vi "sv_Get Audio Weighting Filter Coefficients.vi"(6 "reset filter (F)":bool, 8 "error in (no error)":errorcluster, 9 "weighting filter":T2 items=["Linear", "A-weighting", "B-weighting", "C-weighting", "ITU-R 468-4", "Dolby", "CCITT", "C-message", "Wb", "Wc", "Wd", "We", "Wf", "Wh", "Wj", "Wk", "Wm", "AES17 20 kHz lowpass", "AES17 40 kHz lowpass", "AES17 20 kHz highpass", "AES17 40 kHz highpass"], 11 "scaled signal":waveform(dbl)={"t0"=timestamp(0 s since 1904-01-01), "dt"=0.0, "Y"=[]}) -> (0 "error out":errorcluster, 2 "filter coefficients":T1 {"Forward Coefficients" format="%.4f"; "Reverse Coefficients" format="%.4f"}, 3 "dup scaled signal":waveform(dbl))   [LabVIEW 2017]
doc: "Designs the A, B, or C weighting filter coefficients. The design is based on the ANSI S1.42-1986 standard. This VI also returns the maximum frequency, expressed in hertz, within the tolerance limits based on the selected type (Type 1 or Type 0), according to the ANSI S1.4-1986 standard."
uses:
  <vilib>/addons/_NISVFA/_Shared subVIs/Controls/svc_Weighting Filter Text Ring.ctl
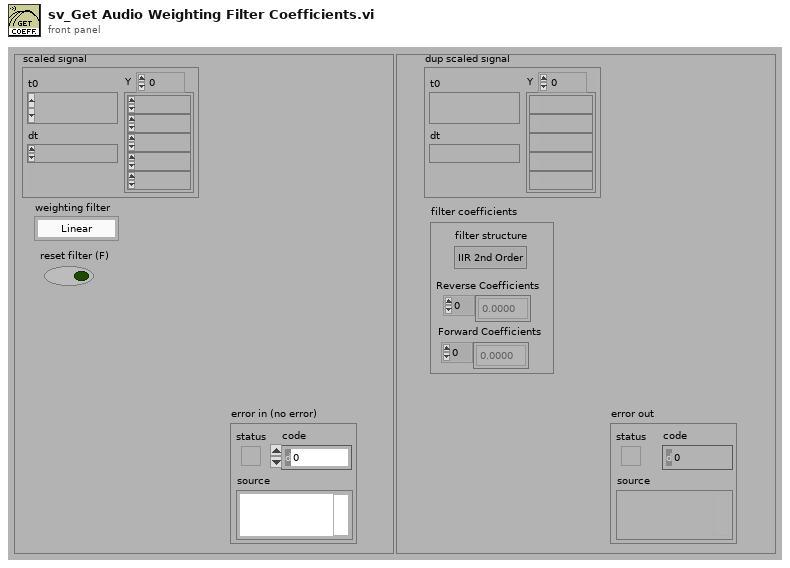
[diagram p1: front panel]
types:
  T1 = cluster{"filter structure":enum32{"IIR 2nd Order", "IIR 4th Order"}, "Reverse Coefficients":dbl[], "Forward Coefficients":dbl[]}
  T2 = typedef "svc_Weighting Filter Text Ring.ctl" = u16
  T3 = cluster{"filter structure":enum32{"IIR 2nd Order", "IIR 4th Order"}, "Reverse Coefficients":dbl[], "Forward Coefficients":dbl[]}[]
  T4 = enum16{"Linear", "A-weighting", "B-weighting", "C-weighting", "ITU-R 468-4", "Dolby", "CCITT", "C-message", "Wb", "Wc", "Wd", "We", "Wf", "Wh", "Wj", "Wk", "Wm", "Undefined"}
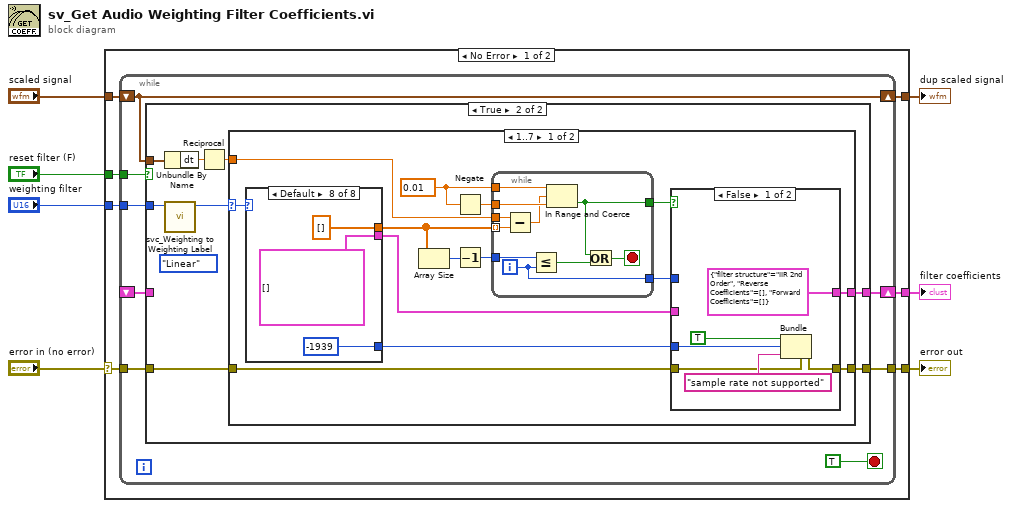
[diagram p0: block diagram]
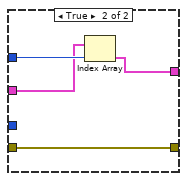
[diagram p3: hidden frame]
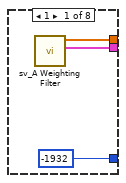
[diagram p4: hidden frame]
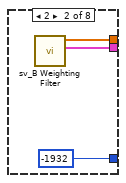
[diagram p5: hidden frame]
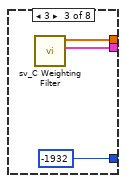
[diagram p6: hidden frame]
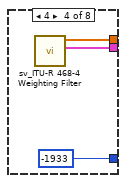
[diagram p7: hidden frame]
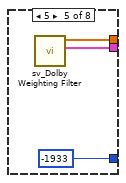
[diagram p8: hidden frame]
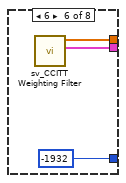
[diagram p9: hidden frame]
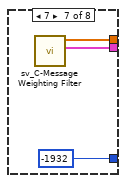
[diagram p10: hidden frame]
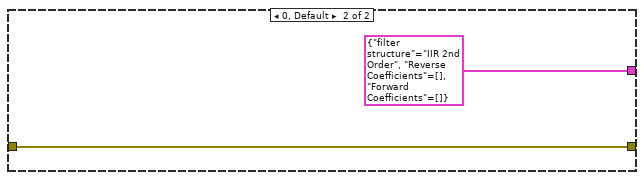
[diagram p11: hidden frame]
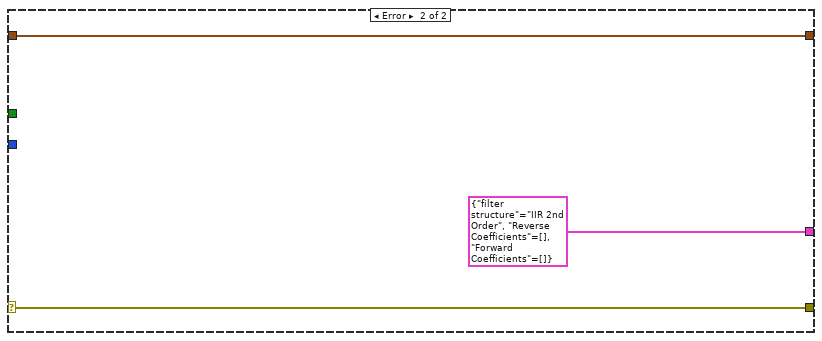
[diagram p12: hidden frame]
diagram:
  n1 = case shown="No Error" "error in (no error)" {
    selector: "error in (no error)" -> [w9 w95]
    tunnel: [w14 T1 {"filter structure"=enum."IIR 2nd Order", "Reverse Coefficients"=[], "Forward Coefficients"=[]} ("filter coefficients")] -> w7
    tunnel: "scaled signal" -> [w12 w94]
    tunnel: [w8 w95] -> w5
    tunnel: [w11 w94] -> w3
    tunnel: "weighting filter" -> [w13 _]
    tunnel: "reset filter (F)" -> [w10 _]
    frame No Error {
      n2 = while {
        tunnel: w13 -> [w21]
        tunnel: w10 -> [w18]
        shift-right: [w22] -> w14
        shift-left: _ -> [w17]
        tunnel: w9 -> [w16]
        tunnel: [w15] -> w8
        shift-right: [w19] -> w11
        shift-left: w12 -> [w19]
        stop <- TRUE stop-if-true
        n3 = case shown="True" w18 {
          tunnel: [w24 w32] -> w22
          tunnel: w21 -> [_ w28]
          tunnel: w19 -> [_ w27]
          tunnel: w17 -> [w24 _]
          tunnel: w16 -> [w23 w26]
          tunnel: [w23 w25] -> w15
          frame False {
          }
          frame True {
            (unwired) T4."Linear" ("weighting enum")
            n4 = Unbundle By Name(w27) -> ("dt"=w31:dbl)
            n5 = call <vilib>:"svc_Weighting to Weighting Label.vi"("weighting filter"=w28) -> ("weighting enum"=w29:T2)  [unwired: 9 in, 1 out]
            n6 = Reciprocal(x=w31) -> (1/x=w30:dbl)
            n7 = case shown="1..7" w29 {
              selector: w29 -> [w46 _]
              tunnel: [w39 T1 {"filter structure"=enum."IIR 2nd Order", "Reverse Coefficients"=[], "Forward Coefficients"=[]} ("filter coefficients")] -> w32
              tunnel: w30 -> [w43 _]
              tunnel: w26 -> [w38 w91]
              tunnel: [w37 w91] -> w25
              frame 1..7 {
                w33 = 0.01
                n8 = case shown="Default" w46 {
                  tunnel: [w69 w72 w75 w78 w81 w84 w87 dbl[] []] -> w36
                  tunnel: [w68 w71 w74 w77 w80 w83 w86 T3 []] -> w35
                  tunnel: [-1932 ("code") -1932 ("code") -1932 ("code") -1933 ("code") -1933 ("code") -1932 ("code") -1932 ("code") -1939 ("code")] -> w34
                  frame 1 {
                    n9 = call <vilib>:"sv_A Weighting Filter.vi"() -> ("time-domain filters at supported sample rates"=w68:T3, "supported sample rates"=w69:dbl[])  [unwired: 10 in]
                  }
                  frame 2 {
                    n10 = call <vilib>:"sv_B Weighting Filter.vi"() -> ("time-domain filters at supported sample rates"=w71:T3, "supported sample rates"=w72:dbl[])  [unwired: 10 in]
                  }
                  frame 3 {
                    n11 = call <vilib>:"sv_C Weighting Filter.vi"() -> ("time-domain filters at supported sample rates"=w74:T3, "supported sample rates"=w75:dbl[])  [unwired: 10 in]
                  }
                  frame 4 {
                    n12 = call <vilib>:"sv_ITU-R 468-4 Weighting Filter.vi"() -> ("time-domain filters at supported sample rates"=w77:T3, "supported sample rates"=w78:dbl[])  [unwired: 8 in, 2 out]
                  }
                  frame 5 {
                    n13 = call <vilib>:"sv_Dolby Weighting Filter.vi"() -> ("time-domain filters at supported sample rates"=w80:T3, "supported sample rates"=w81:dbl[])  [unwired: 8 in, 2 out]
                  }
                  frame 6 {
                    n14 = call <vilib>:"sv_CCITT Weighting Filter.vi"() -> ("time-domain filters at supported sample rates"=w83:T3, "supported sample rates"=w84:dbl[])  [unwired: 8 in, 2 out]
                  }
                  frame 7 {
                    n15 = call <vilib>:"sv_C-Message Weighting Filter.vi"() -> ("time-domain C-message filters at supported sampe rates"=w86:T3, "supported sample rates"=w87:dbl[])  [unwired: 8 in, 2 out]
                  }
                  frame Default {
                  }
                }
                n16 = Array Size(array=w36) -> (size(s)=w45:i32)
                n17 = Negate(x=w33) -> (-x=w42:dbl)
                n18 = Decrement(x=w45) -> (x-1=w44:i32)
                n19 = while {
                  tunnel: w44 -> [w63]
                  tunnel: w43 -> [w66]
                  tunnel: w36 -> [w65] mode=indexing
                  tunnel: w33 -> [w60]
                  tunnel: w42 -> [w59]
                  tunnel: [w61] -> w40
                  tunnel: [w58] -> w41
                  i -> [w61]
                  stop <- w64 stop-if-true
                  n20 = Subtract(x=w66, y=w65) -> (x-y=w57:dbl)
                  n21 = Less Or Equal?(x=w63, y=w61) -> (x <= y?=w62:bool)
                  n22 = In Range and Coerce(upper limit=w60, x=w57, lower limit=w59) -> (In Range?=w58:bool)  [unwired: 1 out]
                  n23 = Or(x=w58, y=w62) -> (x .or. y?=w64:bool)
                }
                n24 = case shown="False" w41 {
                  tunnel: w35 -> [_ w55]
                  tunnel: w40 -> [_ w56]
                  tunnel: [T1 {"filter structure"=enum."IIR 2nd Order", "Reverse Coefficients"=[], "Forward Coefficients"=[]} ("filter coefficients") w54] -> w39
                  tunnel: w38 -> [w48 w53]
                  tunnel: [w49 w53] -> w37
                  tunnel: w34 -> [w51 _]
                  frame False {
                    n25 = Bundle(cluster=w48, "status"=TRUE, "code"=w51, "source"="sample rate not supported") -> (w49:errorcluster)
                  }
                  frame True {
                    n26 = Index Array(array=w55, index=w56) -> (element=w54:T1)
                  }
                }
              }
              frame 0, Default {
              }
            }
          }
        }
      }
    }
    frame Error {
    }
  }
  "filter coefficients" <- w7
  "dup scaled signal" <- w3
  "error out" <- w5
